vi "Pulse Pattern.vi"(2 "width":i32=1, 3 "delay":i32, 4 "amplitude":dbl=1.0 format="%0.2f", 5 "samples":i32=128) -> (0 "error":i32, 1 "Pulse Pattern":dbl[](array[numeric]))   [LabVIEW 2010, in "NI_AALBase.lvlib"]
doc: "Generates an array containing a pulse pattern."
uses:
  NI_AALBase.lvlib
  lvanlys.dll
panel:
  # "Pulse Pattern"
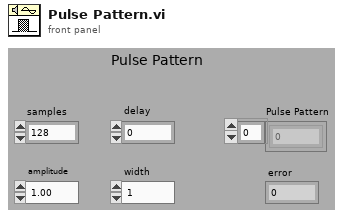
[diagram p1: front panel]
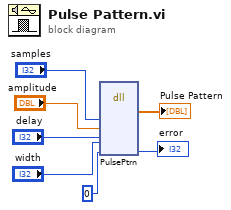
[diagram p0: block diagram]
diagram:
  n1 = dll-call lib="C:/Program Files/National Instruments/LabVIEW 2010/resource/lvanlys.*" fn="PulsePtrn"("samples"="samples", "amplitude"="amplitude", "delay"="delay", "width"="width", 0) -> ("Pulse Pattern"=→"Pulse Pattern":dbl[], →"error":i32)  [unwired: 9 in, 2 out]
